vi "Running.vi"(8 "error in (no error)":errorcluster, 11 "CIFPlugin in":refnum<class "Template_Plugin.lvclass">) -> (0 "error out":errorcluster, 2 "Destroy":bool, 3 "CIFPlugin out":refnum<class "Template_Plugin.lvclass">)   [LabVIEW 2021, in "Template_Plugin.lvclass"]
doc: "This VI is the main execution code. It normally executes with elevated priority. It may be called inside a timed structure to set priority. If it is configured to run outside a timed structure, the priority and execution system can be tuned by changing the settings of this VI."
uses:
  Template_Plugin.lvclass
  C:/Program Files/National Instruments/LabVIEW 2021/vi.lib/CIF Foundation/CIF Core/CIFCore/Class/CIFCorePlugin.lvclass
  <vilib>/CIF Foundation/CIF Core/CIFCore/Class/CIFCorePlugin.lvclass/CIFCorePlugin.ctl
  <vilib>/CIF Foundation/CIF Utilities/Statistics/I64/Stats_I64_CIF_U.lvclass/Stats_I64_CIF_U.ctl
  Template_Plugin.lvclass/Template_Plugin.ctl
  <vilib>/CIF Foundation/CIF Core/Channels/CIFChannelMng/CIFChannelMng.lvclass/CIFChannelMng.ctl
  <vilib>/CIF Foundation/CIF Channels Core/CIFChannels/CIFChannels.lvclass/CIFChannels.ctl
  <vilib>/CIF Foundation/CIF Core/CIFCore/Class/Typedef/Energized States.ctl
  Logic.vi
  <vilib>/CIF Foundation/CIF Core/CIFCore/Class/Accessors/Write Energized State.vi
  <vilib>/CIF Foundation/CIF Core/CIFCore/Class/SubVIs/Timing/Sleep.vi
  <vilib>/CIF Foundation/CIF Core/CIFCore/Class/SubVIs/OOB/Read Core OOB RX.vi
  OOB Comm/Read Comm to Main.vi
  OOB Comm/Send Cyclic to gRPC.vi
  <vilib>/CIF Foundation/CIF Core/CIFCore/Class/Benchmarking/Benchmark Housekeeping.vi
  <vilib>/CIF Foundation/CIF Core/CIFCore/Class/SubVIs/OOB/Update Status from Benchmarks.vi
  <vilib>/CIF Foundation/CIF Core/Channels/CIFChannelMng/Core/Send Channel List Update.vi
  <vilib>/CIF Foundation/CIF Core/CIFCore/Class/SubVIs/OOB/Send Core OOB TX.vi/074d8088-3ad4-4fdc-9542-b009f1b06b72.vi
  <vilib>/CIF Foundation/CIF Utilities/Time/System Time/Sleep Until Future Time.vi
  <vilib>/CIF Foundation/CIF Utilities/Time/System Time/Get System Time.vi
  <vilib>/CIF Foundation/CIF Core/CIFCore/Class/Accessors/Timestamps/Write Execute TS.vi
  <vilib>/Utility/error.llb/Clear Errors.vi
  <vilib>/CIF Foundation/CIF Core/CIFCore/Class/Accessors/Read Sleep Limits (ns).vi
  <vilib>/CIF Foundation/CIF Core/CIFCore/Class/Accessors/Timestamps/Write Target Wake TS.vi
  <vilib>/CIF Foundation/CIF Core/CIFCore/Class/Accessors/Read Plugin Name.vi
  <vilib>/CIF Foundation/CIF Core/CIFCore/Common/Utilities/Add Error.vi
  <vilib>/CIF Foundation/CIF Core/CIFCore/Class/Accessors/Timestamps/Read Running TS.vi
  <vilib>/CIF Foundation/CIF Core/CIFCore/Class/Accessors/Timestamps/Write Sleep TS.vi
  <vilib>/CIF Foundation/CIF Core/CIFCore/Class/Benchmarking/Reset Delay.vi
  <vilib>/CIF Foundation/CIF Core/CIFCore/Class/Accessors/Read Running Internal Data.vi
  <vilib>/CIF Foundation/CIF Core/CIFCore/Class/Accessors/Read Timing Override.vi
  <vilib>/CIF Foundation/CIF Core/CIFCore/Class/Accessors/Read Common Config.vi
  <vilib>/CIF Foundation/CIF Core/CIFCore/Class/Benchmarking/Benchmark Execute.vi
  <vilib>/CIF Foundation/CIF Core/CIFCore/Class/Accessors/Timestamps/Write Housekeeping TS.vi
  <vilib>/CIF Foundation/CIF Core/CIFCore/Class/SubVIs/Refresh Stats.vi
  <vilib>/CIF Foundation/CIF Core/CIFCore/Class/SubVIs/OOB/Receive/Read Clock Map.vi
  <vilib>/CIF Foundation/CIF Core/CIFCore/Class/SubVIs/OOB/Receive/Read Connections.vi
  <vilib>/CIF Foundation/CIF Core/Channels/CIFChannelMng/SubVIs/Connect Channel.vi
  <vilib>/CIF Foundation/CIF Core/CIFCore/Class/SubVIs/OOB/Receive/Read Forces.vi
  <vilib>/CIF Foundation/CIF Core/Channels/CIFChannelMng/SubVIs/Force Channel.vi
  <vilib>/CIF Foundation/CIF Core/Channels/CIFChannelMng/SubVIs/Add FIFO Publisher.vi
  <vilib>/CIF Foundation/CIF Core/CIFCore/Class/SubVIs/OOB/Receive/Read Publisher Instance.vi
  <vilib>/CIF Foundation/CIF Core/Channels/CIFChannelMng/Core/Send Publisher Instance Return.vi
  <vilib>/CIF Foundation/CIF Core/Channels/CIFChannelMng/SubVIs/Remove FIFO Publisher.vi
  <vilib>/CIF Foundation/CIF Core/CIFCore/Class/SubVIs/OOB/Read Core OOB RX.vi/a31a91a9-4107-4750-8e0d-44486e9a3a34.vi
  OOB Comm/Read Comm to Main.vi/4efb0375-f1de-4191-b03f-44d34e6646cb.vi
  OOB Comm/Read Comm to Main.vi/525c214c-2a6b-4e7b-b3ce-0ad96b412d2f.vi
  OOB Comm/Send Cyclic to gRPC.vi/0c0f428d-7269-422d-ba27-f9d6fa7232ec.vi
  <vilib>/CIF Foundation/CIF Core/CIFCore/Class/Accessors/Read Refresh.vi
  <vilib>/CIF Foundation/CIF Utilities/Statistics/I64/X1 minus X0.vi
  <vilib>/CIF Foundation/CIF Core/CIFCore/Class/Accessors/Timestamps/Read Housekeeping TS.vi
  <vilib>/CIF Foundation/CIF Utilities/Statistics/I64/Get Stats.vi
  <vilib>/CIF Foundation/CIF Core/Channels/CIFChannelMng/Core/Send Channel List Update.vi/463ebf4c-8748-40f9-8ad3-9e61c16a01a6.vi
  <vilib>/CIF Foundation/CIF CIPC/SubVIs/Check Error.vi
  <vilib>/CIF Foundation/CIF CIPC/SubVIs/Notify Of New Write.vi
  <vilib>/CIF Foundation/CIF CIPC/SubVIs/Get dll Path.vi
  <vilib>/CIF Foundation/CIF CIPC/SubVIs/Get Element Write Position.vi
  <vilib>/CIF Foundation/CIF Utilities/Time/SubVIs/Add Error.vi
  <vilib>/CIF Foundation/CIF Utilities/Time/System Time/LabVIEW Time to TAI Time.vi
  <vilib>/CIF Foundation/CIF Utilities/Errors/Append Error Location.vi
  <vilib>/CIF Foundation/CIF Utilities/Statistics/I64/Cyclic.vi
  <vilib>/CIF Foundation/CIF Core/CIFCore/Class/Accessors/Timestamps/Read Execute TS.vi
  <vilib>/CIF Foundation/CIF Core/CIFCore/Class/Accessors/Timestamps/Read Sleep TS.vi
  <vilib>/CIF Foundation/CIF Core/CIFCore/Class/Accessors/Timestamps/Read Target Wake TS.vi
  <vilib>/CIF Foundation/CIF Core/Channels/CIFChannelMng/Utilities/Get Channel Index by Name.vi
  <vilib>/CIF Foundation/CIF Channels Core/CIFChannels/Accessors/Read Channel State.vi
  <vilib>/CIF Foundation/CIF Channels Core/CIFChannels/Accessors/Read Tag Forced.vi
  <vilib>/CIF Foundation/CIF Core/Channels/CIFChannelMng/SubVIs/Add Error Channel Manager.vi
  <vilib>/CIF Foundation/CIF Core/Channels/CIFChannelMng/Core/Send Publisher Instance Return.vi/9db40550-ae0b-4108-a32d-02e81b824dbe.vi
  <vilib>/CIF Foundation/CIF Core/Channels/CIFChannelMng/SubVIs/Get Original FIFO Channel Name.vi
  <vilib>/CIF Foundation/CIF CIPC/SubVIs/Wait For N Elements Available.vi
  <vilib>/CIF Foundation/CIF CIPC/SubVIs/Get Element Read Position.vi
  <vilib>/CIF Foundation/CIF CIPC/SubVIs/Set Element Read Position.vi
  <vilib>/CIF Foundation/CIF Utilities/Statistics/I64/X1 minus X0.vi/dfabcf33-0dbc-4041-80a5-3dc0c86d2989.vi
  <vilib>/CIF Foundation/CIF Utilities/Statistics/I64/Cyclic.vi/dfabcf33-0dbc-4041-80a5-3dc0c86d2989.vi
  <vilib>/CIF Foundation/CIF Channels Core/ChannelCommon/Utilities/Add Error.vi
  <vilib>/CIF Foundation/CIF Utilities/Statistics/I64/X1 minus X0.vi/dfabcf33-0dbc-4041-80a5-3dc0c86d2989.vi/9eb60a9a-770f-4d2d-8b3f-8465c267ecc9.vi
  <vilib>/CIF Foundation/CIF Utilities/Statistics/I64/Cyclic.vi/dfabcf33-0dbc-4041-80a5-3dc0c86d2989.vi/9eb60a9a-770f-4d2d-8b3f-8465c267ecc9.vi
  <vilib>/CIF Foundation/CIF CIPC/SubVIs/Get Element Info Variant.vi
  <vilib>/Utility/error.llb/Trim Whitespace.vi
  <vilib>/Utility/error.llb/Error Cluster From Error Code.vi
  <vilib>/CIF Foundation/CIF Channels Core/CIFChannels/Core/Set Force.vi
  <vilib>/CIF Foundation/CIF Core/CIFCore/Class/CIFCorePlugin.lvclass
  <vilib>/CIF Foundation/CIF Channels Core/CIFChannels/CIFChannels.lvclass
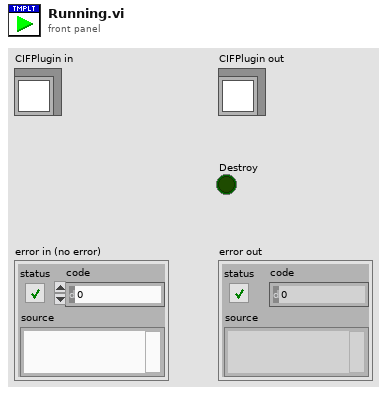
[diagram p1: front panel]
types:
  T1 = typedef "CIFCorePlugin.lvclass/Energized States.ctl" = enum16{"Listen", "Prepare", "Execute", "Housekeep", "Cleanup", "Destroy"}
  T2 = typedef "CIFCorePlugin.lvclass/Running State Logic.ctl" = enum16{"Execute", "Housekeep", "Cleanup", "Error", "Destroy"}
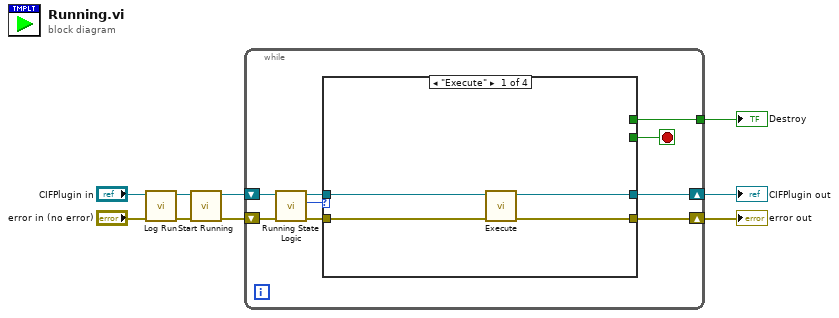
[diagram p0: block diagram]
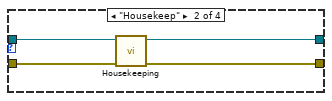
[diagram p2: hidden frame]
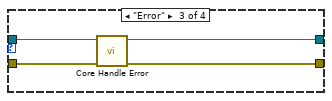
[diagram p3: hidden frame]
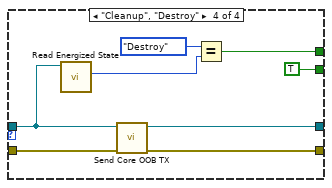
[diagram p4: hidden frame]
diagram:
  n1 = call <vilib>:"Log Run.vi"("error in (no error)"="error in (no error)", "CIFCorePlugin in"="CIFPlugin in") -> ("error out"=w8:errorcluster, "CIFCorePlugin out"=w9:refnum<class "Template_Plugin.lvclass">)  [unwired: 8 in]
  n2 = call <vilib>:"Start Running.vi"("error in (no error)"=w8, "CIFCorePlugin in"=w9) -> ("error out"=w7:errorcluster, "CIFCorePlugin out"=w6:refnum<class "Template_Plugin.lvclass">)  [unwired: 8 in]
  n3 = while {
    shift-right: [w13] -> w2
    shift-left: w6 -> [w18]
    shift-right: [w12] -> w1
    shift-left: w7 -> [w17]
    tunnel: [w10] -> w3
    stop <- w11 stop-if-true
    n4 = call <vilib>:"Running State Logic.vi"("error in (no error)"=w17, "CIFCorePlugin in"=w18) -> ("error out"=w14:errorcluster, "Running State Logic"=w16:T2, "CIFCorePlugin out"=w15:refnum<class "Template_Plugin.lvclass">)  [unwired: 7 in]
    n5 = case shown="\"Execute\"" w16 {
      tunnel: w15 -> [w22 w26 w30 w32]
      tunnel: w14 -> [w21 w25 w29 w37]
      tunnel: [w20 w24 w28 w36] -> w13
      tunnel: [w19 w23 w27 w35] -> w12
      tunnel: [_ _ _ TRUE] -> w11
      tunnel: [_ _ _ w33] -> w10
      frame "Execute" {
        n6 = call "Execute.vi"("error in (no error)"=w21, "CIFPlugin in"=w22) -> ("error out"=w19:errorcluster, "CIFPlugin out"=w20:refnum<class "Template_Plugin.lvclass">)  [unwired: 8 in]
      }
      frame "Housekeep" {
        n7 = call "Housekeeping.vi"("error in (no error)"=w25, "CIFPlugin in"=w26) -> ("error out"=w23:errorcluster, "CIFPlugin out"=w24:refnum<class "Template_Plugin.lvclass">)  [unwired: 8 in]
      }
      frame "Error" {
        n8 = call <vilib>:"Core Handle Error.vi"("error in (no error)"=w29, "CIFTemplateNode in"=w30) -> ("error out"=w27:errorcluster, "CIFTemplateNode out"=w28:refnum<class "Template_Plugin.lvclass">)  [unwired: 8 in]
      }
      frame "Cleanup", "Destroy" {
        n9 = call <vilib>:"Read Energized State.vi"("CIFCorePlugin in"=w32) -> ("Energized State"=w31:T1)  [unwired: 8 in, 2 out]
        n10 = call <vilib>:"Send Core OOB TX.vi"("error in (no error)"=w37, "CIFCorePlugin in"=w32) -> ("error out"=w35:errorcluster, "CIFCorePlugin out"=w36:refnum<class "Template_Plugin.lvclass">)  [unwired: 8 in]
        n11 = Equal?(x=Energized_States."Destroy", y=w31) -> (x = y?=w33:bool)
      }
    }
  }
  "error out" <- w1
  "Destroy" <- w3
  "CIFPlugin out" <- w2
